vi "append line ending (sub-vi).vi"(1 "line ending (\\r\\n)":string="\r\n", 2 "string in":string) -> (7 "string out":string)   [LabVIEW 2021]
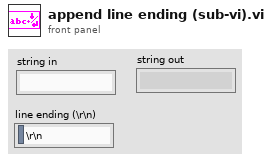
[diagram p1: front panel]
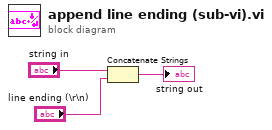
[diagram p0: block diagram]
diagram:
  n1 = Concatenate Strings("string in", "line ending (\\r\\n)") -> (→"string out":string)
